vi "Set Timer (Core).vi"(5 "Quick Timer":T4 {"Set-Time (s)" format="%<%H:%M>t"}, 6 "Start/End Timer":T1 {"Start-Date (s)" format="%<%Y/%m/%d>T"; "Start-Time (s)" format="%<%H:%M>t"}, 7 "Timer Number":T5, 8 "error in (no error)":errorcluster, 10 "Address (0)":i32, 11 "VISA resource name":refnum<visa-resource-name>) -> (0 "error out":errorcluster, 1 "NACK":bool, 2 "ACK":bool, 3 "VISA resource name out":refnum<visa-resource-name>, 4 "Error":bool)   [LabVIEW 2016, in "Environment Chamber.lvlib" / "Climatic Chamber.lvlib"]
doc: "<b>Timer writing</B>\n\nEdits the quick timer, start timer or end timer."
uses:
  Climatic Chamber.lvlib
  Private/Type Defs/TimerNumber Enum.ctl
  Private/Type Defs/QuickTimer Cluster.ctl
  Private/Type Defs/Operation_Stop Mode Enum.ctl
  Private/Type Defs/Start_End Timer Cluster.ctl
  Private/Type Defs/Start Mode Enum.ctl
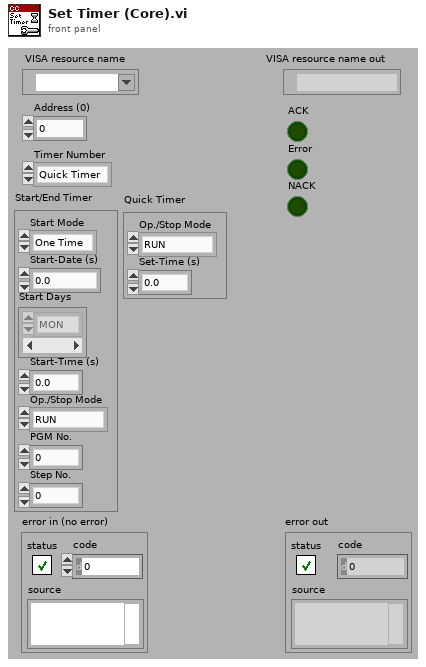
[diagram p1: front panel]
types:
  T1 = typedef "Environment Chamber.lvlib/Climatic Chamber.lvlib/Start_End Timer Cluster.ctl" = cluster{"Start Mode":T2, "Start-Date (s)":dbl, "Start Days":enum16{"MON", "TUE", "WED", "THU", "FRI", "SAT", "SUN"}[], "Start-Time (s)":dbl, "Op./Stop Mode":T3, "PGM No.":i32, "Step No.":i32}
  T2 = typedef "Environment Chamber.lvlib/Climatic Chamber.lvlib/Start Mode Enum.ctl" = enum16{"One Time", "Weekly", "Daily"}
  T3 = typedef "Environment Chamber.lvlib/Climatic Chamber.lvlib/Operation_Stop Mode Enum.ctl" = enum16{"RUN", "CONSTANT", "STANDBY", "OFF"}
  T4 = typedef "Environment Chamber.lvlib/Climatic Chamber.lvlib/QuickTimer Cluster.ctl" = cluster{"Op./Stop Mode":T3, "Set-Time (s)":dbl}
  T5 = typedef "Environment Chamber.lvlib/Climatic Chamber.lvlib/TimerNumber Enum.ctl" = enum16{"Quick Timer", "Start Timer", "End Timer"}
  T6 = enum16{"MON", "TUE", "WED", "THU", "FRI", "SAT", "SUN"}[]
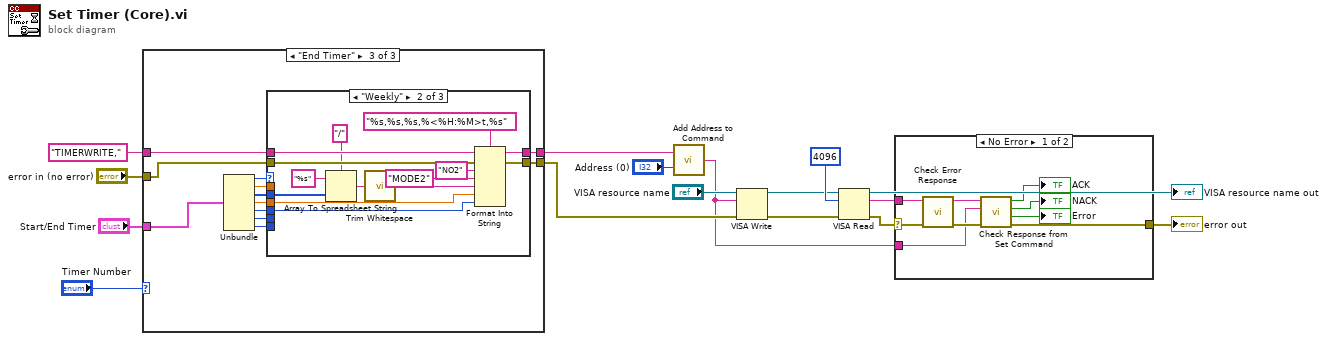
[diagram p0: block diagram]
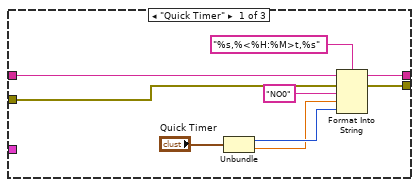
[diagram p2: hidden frame]
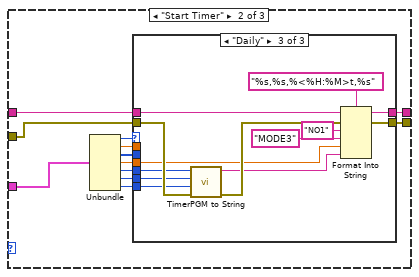
[diagram p3: hidden frame]
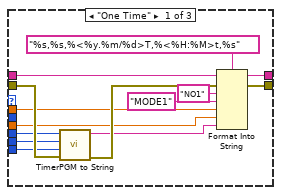
[diagram p4: hidden frame]
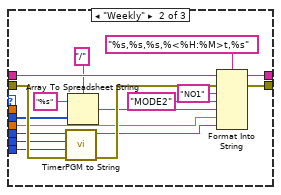
[diagram p5: hidden frame]
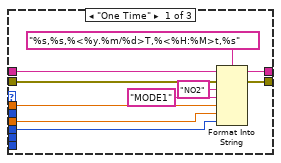
[diagram p6: hidden frame]
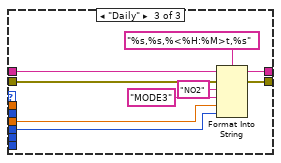
[diagram p7: hidden frame]
diagram:
  n1 = case shown="\"End Timer\"" "Timer Number" {
    tunnel: "TIMERWRITE," -> [w25 w36 w92]
    tunnel: [w24 w34 w90] -> w2
    tunnel: "error in (no error)" -> [w23 w35 w91]
    tunnel: [w22 w37 w93] -> w16
    tunnel: "Start/End Timer" -> [_ w26 w82]
    frame "Quick Timer" {
      n2 = Unbundle("Quick Timer") -> ("Op./Stop Mode"=w19:T3, "Set-Time (s)"=w18:dbl)
      n3 = Format Into String(format string="%s,%<%H:%M>t,%s", initial string=w25, error in=w23, "NO0" ("input 1"), w18, w19) -> (resulting string=w24:string, error out=w22:errorcluster)
    }
    frame "Start Timer" {
      n4 = Unbundle(w26) -> ("Start Mode"=w30:T2, "Start-Date (s)"=w33:dbl, "Start Days"=w27:T6, "Start-Time (s)"=w32:dbl, "Op./Stop Mode"=w31:T3, "PGM No."=w29:i32, "Step No."=w28:i32)
      n5 = case shown="\"Daily\"" w30 {
        tunnel: [w49 w66 w79] -> w37
        tunnel: w36 -> [w48 w65 w78]
        tunnel: w35 -> [w51 w67 w80]
        tunnel: [w47 w64 w77] -> w34
        tunnel: w33 -> [w44 _ _]
        tunnel: w32 -> [w43 w61 w73]
        tunnel: w31 -> [w41 w55 w72]
        tunnel: w29 -> [w40 w54 w71]
        tunnel: w28 -> [w39 w53 w70]
        tunnel: w27 -> [_ w59 _]
        frame "One Time" {
          n6 = call "TimerPGM to String.vi"("error in"=w51, "Step No."=w39, "PGM No."=w40, "Op./Stop Mode"=w41) -> ("error out"=w50:errorcluster, "String out"=w38:string)  [unwired: 6 in]
          n7 = Format Into String(format string="%s,%s,%<%y.%m/%d>T,%<%H:%M>t,%s", initial string=w48, error in=w50, "NO1" ("input 1"), "MODE1" ("input 1"), w44, w43, w38) -> (resulting string=w47:string, error out=w49:errorcluster)
        }
        frame "Weekly" {
          n8 = call "TimerPGM to String.vi"("error in"=w67, "Step No."=w53, "PGM No."=w54, "Op./Stop Mode"=w55) -> ("error out"=w68:errorcluster, "String out"=w52:string)  [unwired: 6 in]
          n9 = Array To Spreadsheet String(delimiter (Tab)="/", array=w59, 3:"%s" ("format string")) -> (spreadsheet string=w56:string)
          n10 = Format Into String(format string="%s,%s,%s,%<%H:%M>t,%s", initial string=w65, error in=w68, "NO1" ("input 1"), "MODE2" ("input 1"), w56, w61, w52) -> (resulting string=w64:string, error out=w66:errorcluster)
        }
        frame "Daily" {
          n11 = call "TimerPGM to String.vi"("error in"=w80, "Step No."=w70, "PGM No."=w71, "Op./Stop Mode"=w72) -> ("error out"=w81:errorcluster, "String out"=w69:string)  [unwired: 6 in]
          n12 = Format Into String(format string="%s,%s,%<%H:%M>t,%s", initial string=w78, error in=w81, "NO1" ("input 1"), "MODE3" ("input 1"), w73, w69) -> (resulting string=w77:string, error out=w79:errorcluster)
        }
      }
    }
    frame "End Timer" {
      n13 = Unbundle(w82) -> ("Start Mode"=w86:T2, "Start-Date (s)"=w89:dbl, "Start Days"=w83:T6, "Start-Time (s)"=w88:dbl, "Op./Stop Mode"=w87:T3, "PGM No."=w85:i32, "Step No."=w84:i32)
      n14 = case shown="\"Weekly\"" w86 {
        tunnel: [w103 w117 w126] -> w93
        tunnel: w92 -> [w102 w116 w125]
        tunnel: w91 -> [w101 w115 w124]
        tunnel: [w100 w114 w123] -> w90
        tunnel: w89 -> [w97 _ _]
        tunnel: w88 -> [w96 w111 w119]
        tunnel: w87 -> [w95 w110 w118]
        tunnel: w85 -> [_ _ _]
        tunnel: w84 -> [_ _ _]
        tunnel: w83 -> [_ w108 _]
        frame "One Time" {
          n15 = Format Into String(format string="%s,%s,%<%y.%m/%d>T,%<%H:%M>t,%s", initial string=w102, error in=w101, "NO2" ("input 1"), "MODE1" ("input 1"), w97, w96, w95) -> (resulting string=w100:string, error out=w103:errorcluster)
        }
        frame "Weekly" {
          n16 = Array To Spreadsheet String(delimiter (Tab)="/", array=w108, 3:"%s" ("format string")) -> (spreadsheet string=w105:string)
          n17 = call <vilib>:"Trim Whitespace.vi"("string"=w105) -> ("trimmed string"=w104:string)  [unwired: 1 in]
          n18 = Format Into String(format string="%s,%s,%s,%<%H:%M>t,%s", initial string=w116, error in=w115, "NO2" ("input 1"), "MODE2" ("input 1"), w104, w111, w110) -> (resulting string=w114:string, error out=w117:errorcluster)
        }
        frame "Daily" {
          n19 = Format Into String(format string="%s,%s,%<%H:%M>t,%s", initial string=w125, error in=w124, "NO2" ("input 1"), "MODE3" ("input 1"), w119, w118) -> (resulting string=w123:string, error out=w126:errorcluster)
        }
      }
    }
  }
  n20 = call "Add Address to Command.vi"("Address (0)"="Address (0)", "Command"=w2) -> ("Command OUT"=w6:string)
  n21 = VISA Write(VISA resource name="VISA resource name", write buffer=w6, error in (no error)=w16) -> (VISA resource name out=w13:refnum<visa-resource-name>, error out=w12:errorcluster)  [unwired: 1 out]
  n22 = VISA Read(VISA resource name=w13, byte count=u32 4096, error in (no error)=w12) -> (VISA resource name out=→"VISA resource name out":refnum<visa-resource-name>, read buffer=w8:string, error out=w9:errorcluster)  [unwired: 1 out]
  n23 = case shown="No Error" w9 {
    selector: w9 -> [w134 w136]
    tunnel: w8 -> [w135 _]
    tunnel: [w130 w136] -> w7
    tunnel: w6 -> [w131 _]
    frame No Error {
      n24 = call "Check Error Response.vi"("error in (no error)"=w134, "read String"=w135) -> ("error out"=w133:errorcluster, "String out"=w132:string)  [unwired: 7 in, 1 out]
      n25 = call "Check Response from Set Command.vi"("error in (no error)"=w133, "Command"=w131, "Response"=w132) -> ("error out"=w130:errorcluster, "Error"=→"Error":bool, "NACK"=→"NACK":bool, "ACK"=→"ACK":bool)  [unwired: 5 in]
    }
    frame Error {
    }
  }
  "error out" <- w7
